vi "[NameData] - Strings from Variants.vi"(4 "Format Cluster":T2, 6 "String Format Select":T1, 7 "Section Name (Name Of \"Anything\")":string, 8 "Error":errorcluster, 9 "Remove Source name":bool, 11 "Anything":variant) -> (0 "Error Out":errorcluster, 2 "Values Out":string[](array[string]), 3 "Names Out":string[](array[string]), 5 "Section Out":string)   [LabVIEW 2015]
uses:
  TypeDefs_Utility/Cluster_NameData_String Format Data.ctl
  TypeDefs_Utility/ENUM_NameData_String Format Select.ctl
  <vilib>/Utility/VariantDataType/VariantType.lvlib
panel:
  # "%.2f %g %e %p"
  # "%d %h %o %b"
  # "'%s'"
  # "%x %X"
  # "True,False -1,0 Yes,No"
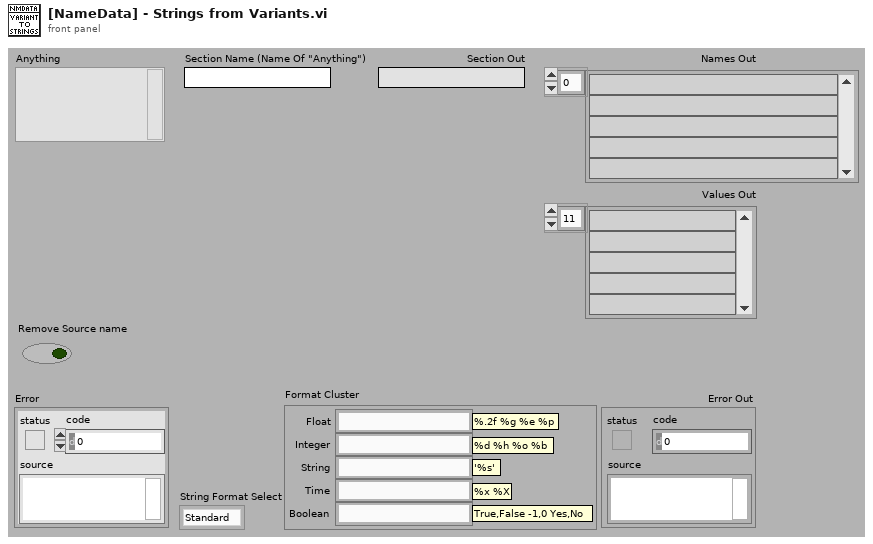
[diagram p1: front panel]
types:
  T1 = typedef "ENUM_NameData_String Format Select.ctl" = enum16{"Standard", "Access DB", "Custom"}
  T2 = typedef "Cluster_NameData_String Format Data.ctl" = cluster{"Float":string, "Integer":string, "String":string, "Time":string, "Boolean":string}
  T3 = typedef "VariantType.lvlib/Type.ctl" = enum8{"Invalid Type", "Void", "I8", "I16", "I32", "I64", "U8", "U16", "U32", "U64", "Single Float", "Double Float", "Extended Float", "Single Complex", "Double Complex", "Extended Complex", "Enum U8", "Enum U16", "Enum U32", "Enum U64", "Single Float With Unit", "Double Float With Unit", "Extended Float With Unit", "Single Complex with Unit", "Double Complex with Unit", "Extended Complex with Unit", "Boolean", "String", "Path", "Picture", "Tag", "Array", "Cluster", "Variant", "LV Variant", "Waveform", "Timestamp", "Digital Waveform", "Digital Data", "ExpressData", "Refnum", "External Data", "VI", "Poly VI", "LabVIEW Class Instance", "Fixed Point"}
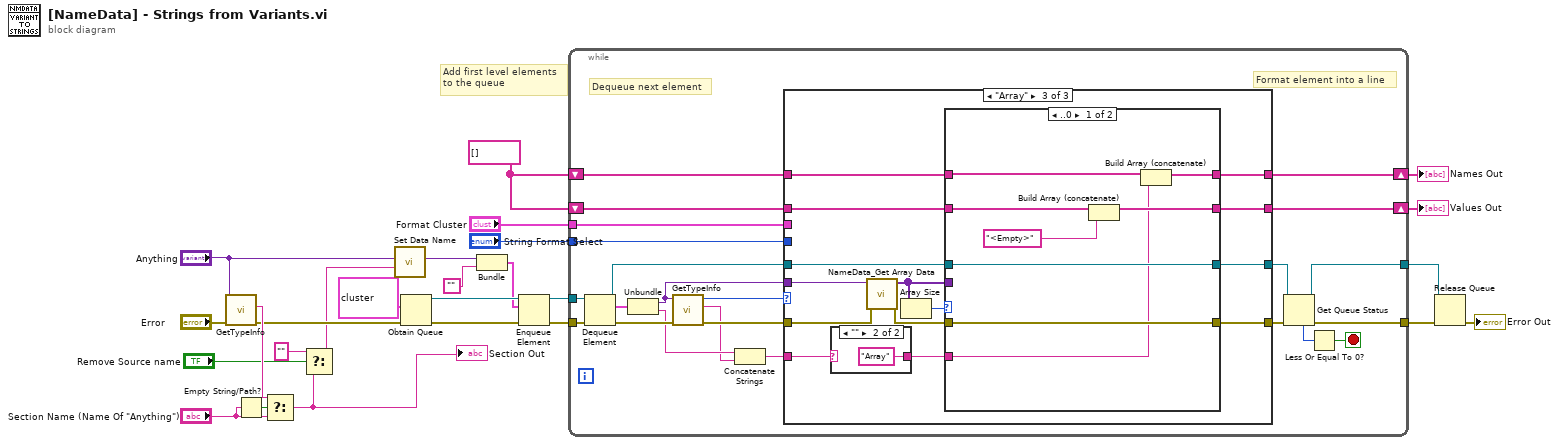
[diagram p0: block diagram]
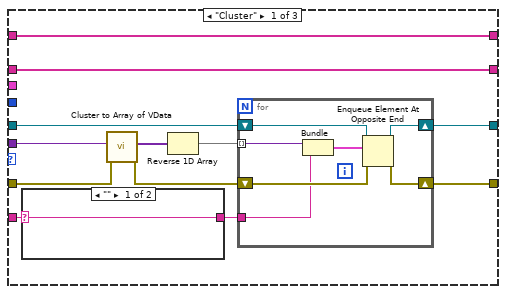
[diagram p2: hidden frame]
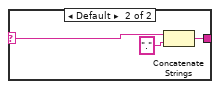
[diagram p3: hidden frame]
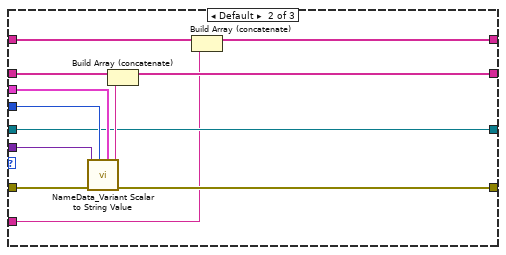
[diagram p4: hidden frame]
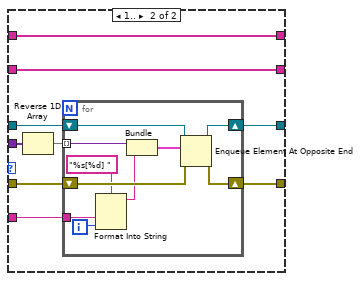
[diagram p6: hidden frame]
diagram:
  w13 = string[] []
  # "Add first level elements\nto the queue"
  n1 = call <vilib>:"GetTypeInfo.vi"("error in (no error)"="Error", "Variant"="Anything") -> ("error out"=w8:errorcluster, "Name"=w17:string)  [unwired: 5 in, 3 out]
  n2 = Empty String/Path?(string/path="Section Name (Name Of \"Anything\")") -> (empty?=w18:bool)
  n3 = Select(t=w17, s=w18, f="Section Name (Name Of \"Anything\")") -> (s? t:f=w2:string)
  "Section Out" <- w2
  n4 = Select(t="", s="Remove Source name", f=w2) -> (s? t:f=w3:string)
  n5 = call "Set Data Name.vi"("Data Name"=w3, "Data"="Anything") -> ("Renamed Data"=w5:variant)  [unwired: 8 in, 1 out]
  n6 = Obtain Queue(element data type=cluster{"Variant":variant, "Name":string} {"Variant"=variant, "Name"=""}, error in (no error)=w8) -> (queue out=w26:refnum<queue>, error out=w25:errorcluster)  [unwired: 3 in, 1 out]
  n7 = Bundle("Renamed Data"=w5, "") -> (w15:cluster{"Renamed Data":variant, string})  [unwired: 1 in]
  n8 = Enqueue Element(queue=w26, element=w15, error in (no error)=w25) -> (queue out=w23:refnum<queue>, error out=w24:errorcluster)  [unwired: 1 in, 1 out]
  n9 = while {
    tunnel: w24 -> [w49]
    tunnel: [w46] -> w22
    tunnel: w23 -> [w47]
    tunnel: [w43] -> w21
    shift-right: [w35] -> w9
    shift-left: w13 -> [w30]
    shift-right: [w34] -> w10
    shift-left: w13 -> [w31]
    tunnel: "Format Cluster" -> [w29]
    tunnel: "String Format Select" -> [w28]
    stop <- w44 stop-if-true
    # "Format element into a line"
    # "Dequeue next element"
    n10 = Dequeue Element(queue=w47, error in (no error)=w49) -> (queue out=w41:refnum<queue>, element=w39:cluster{"Variant":variant, "Name":string}, error out=w48:errorcluster)  [unwired: 1 in, 1 out]
    n11 = Unbundle(w39) -> ("Variant"=w38:variant, "Name"=w37:string)
    n12 = call <vilib>:"GetTypeInfo.vi"("error in (no error)"=w48, "Variant"=w38) -> ("error out"=w36:errorcluster, "Name"=w27:string, "Type Enum"=w32:T3)  [unwired: 5 in, 2 out]
    n13 = Concatenate Strings(w37, w27) -> (w33:string)
    n14 = case shown="\"Array\"" w32 {
      tunnel: [w61 w74 w95] -> w42
      tunnel: w41 -> [w60 w74 w96]
      tunnel: [w59 w84 w93] -> w40
      tunnel: w38 -> [w58 w77 w97]
      tunnel: w36 -> [w57 w78 w98]
      tunnel: [w51 w81 w89] -> w35
      tunnel: [w52 w82 w88] -> w34
      tunnel: w33 -> [w50 w73 w86]
      tunnel: w31 -> [w52 w83 w91]
      tunnel: w30 -> [w51 w80 w90]
      tunnel: w29 -> [_ w75 _]
      tunnel: w28 -> [_ w76 _]
      frame "Cluster" {
        n15 = case shown="\"\"" w50 {
          selector: w50 -> [w62 w63]
          tunnel: [w62 w64] -> w53
          frame "" {
          }
          frame Default {
            n16 = Concatenate Strings(w63, "." ("string")) -> (w64:string)
          }
        }
        n17 = call "Cluster to Array of VData.vi"("error in (no error)"=w57, "Cluster"=w58) -> ("error out"=w55:errorcluster, "Array of VData"=w54:variant[])  [unwired: 8 in]
        n18 = Reverse 1D Array(array=w54) -> (reversed array=w56:variant[])
        n19 = for {
          tunnel: w56 -> [w67] mode=indexing
          tunnel: w53 -> [w66]
          shift-right: [w69] -> w61
          shift-left: w60 -> [w72]
          shift-right: [w70] -> w59
          shift-left: w55 -> [w71]
          n20 = Bundle("Variant"=w67, w66) -> (w68:cluster{"Variant":variant, string})  [unwired: 1 in]
          n21 = Enqueue Element At Opposite End(queue=w72, element=w68, error in (no error)=w71) -> (queue out=w69:refnum<queue>, error out=w70:errorcluster)  [unwired: 1 in, 1 out]
        }
      }
      frame Default {
        n22 = call "NameData_Variant Scalar to String Value.vi"("Format Cluster"=w75, "String Format Select"=w76, "Error"=w78, "Variant"=w77) -> ("Error Out"=w84:errorcluster, "Value Out"=w79:string)  [unwired: 5 in, 1 out]
        n23 = Build Array (concatenate)(w80, w79) -> (w81:string[])
        n24 = Build Array (concatenate)(w83, w73) -> (w82:string[])
      }
      frame "Array" {
        n25 = case shown="\"\"" w86 {
          selector: w86 -> [w99 _]
          tunnel: [w99 "Array"] -> w85
          frame Default {
          }
          frame "" {
          }
        }
        n26 = call "NameData_Get Array Data.vi"("Error"=w98, "Array Variant"=w97) -> ("Error Out"=w94:errorcluster, "Data Array Out"=w92:variant[])  [unwired: 7 in, 1 out]
        n27 = Array Size(array=w92) -> (size(s)=w87:i32)
        n28 = case shown="..0" w87 {
          tunnel: w96 -> [w103 w117]
          tunnel: [w103 w116] -> w95
          tunnel: w85 -> [w101 w115]
          tunnel: w94 -> [w102 w114]
          tunnel: [w102 w113] -> w93
          tunnel: w92 -> [_ w111]
          tunnel: w91 -> [w108 w109]
          tunnel: w90 -> [w106 w110]
          tunnel: [w105 w110] -> w89
          tunnel: [w107 w109] -> w88
          frame ..0 {
            n29 = Build Array (concatenate)(w106, "<Empty>") -> (w105:string[])
            n30 = Build Array (concatenate)(w108, w101) -> (w107:string[])
          }
          frame 1.. {
            n31 = Reverse 1D Array(array=w111) -> (reversed array=w112:variant[])
            n32 = for {
              tunnel: w112 -> [w122] mode=indexing
              tunnel: w115 -> [w120]
              shift-right: [w124] -> w116
              shift-left: w117 -> [w127]
              shift-right: [w125] -> w113
              shift-left: w114 -> [w126]
              i -> [w119]
              n33 = Format Into String(format string="%s[%d] ", w120, w119) -> (resulting string=w118:string)  [unwired: 2 in, 1 out]
              n34 = Bundle("Variant"=w122, w118) -> (w123:cluster{"Variant":variant, string})  [unwired: 1 in]
              n35 = Enqueue Element At Opposite End(queue=w127, element=w123, error in (no error)=w126) -> (queue out=w124:refnum<queue>, error out=w125:errorcluster)  [unwired: 1 in, 1 out]
            }
          }
        }
      }
    }
    n36 = Get Queue Status(queue=w42, error in (no error)=w40) -> (queue out=w43:refnum<queue>, error out=w46:errorcluster, # elements in queue=w45:i32)  [unwired: 1 in, 5 out]
    n37 = Less Or Equal To 0?(x=w45) -> (x <= 0?=w44:bool)
  }
  "Names Out" <- w10
  "Values Out" <- w9
  n38 = Release Queue(queue=w21, error in (no error)=w22) -> (error out=→"Error Out":errorcluster)  [unwired: 1 in, 2 out]
